vi "SaveImg.vi"(0 "零件型号":string, 1 "Image":T1, 2 "Fold路径":path) -> ()   [LabVIEW 2014]
uses:
  <vilib>/vision/Image Controls.llb/IMAQ Image.ctl
panel:
  out "添加的路径":path
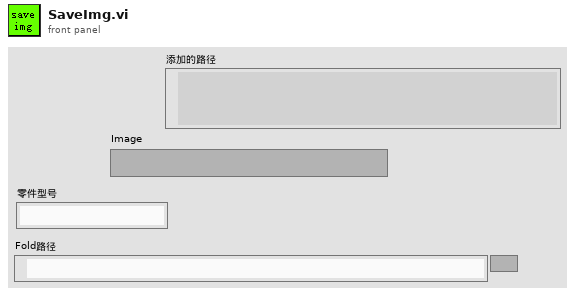
[diagram p1: front panel]
types:
  T1 = typedef "IMAQ Image.ctl" = refnum<image>
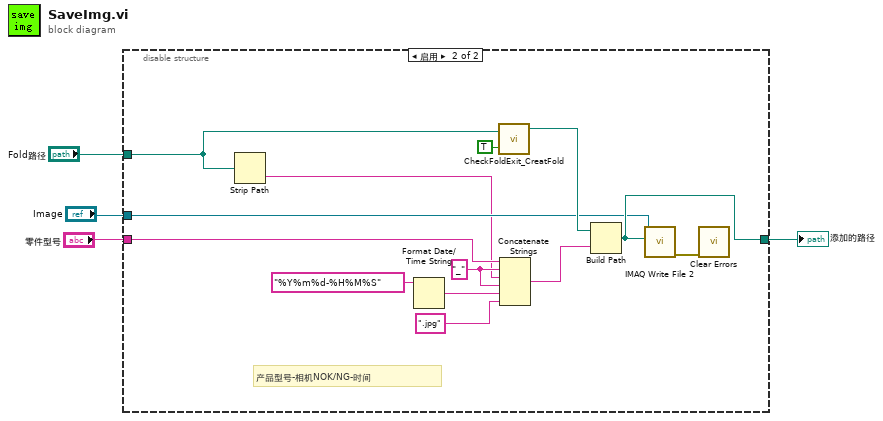
[diagram p0: block diagram]
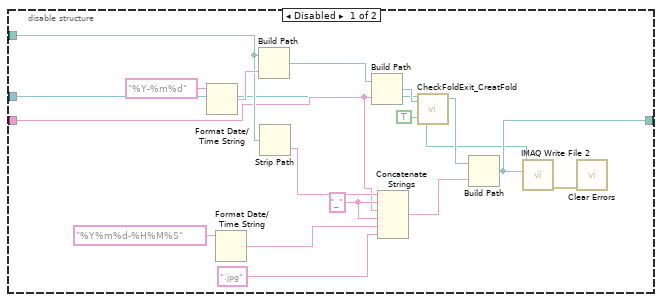
[diagram p2: hidden frame]
diagram:
  n1 = disable-structure shown="启用" {
    disable-tunnel: [w18 w26] -> w4
    disable-tunnel: "Fold路径" -> [w9 w22]
    disable-tunnel: "零件型号" -> [w6 w24]
    disable-tunnel: "Image" -> [w5 w25]
    frame Disabled {
      w7 = "_" ("字符串")
      n2 = Format Date/Time String(time format string (%c)="%Y-%m%d") -> (date/time string=w21:string)  [unwired: 2 in]
      n3 = Format Date/Time String(time format string (%c)="%Y%m%d-%H%M%S") -> (date/time string=w16:string)  [unwired: 2 in]
      n4 = Build Path(base path=w9, name or relative path=w21) -> (appended path=w10:path)
      n5 = Strip Path(path=w9) -> (name=w8:string)  [unwired: 1 out]
      n6 = Build Path(base path=w10, name or relative path=w6) -> (appended path=w12:path)
      n7 = Concatenate Strings(w8, w7, w6, w7, w16, ".jpg" ("string")) -> (w17:string)
      n8 = call "CheckFoldExit_CreatFold.vi"("path in"=w12, "FoldOrFile¡H"=TRUE) -> ("File out"=w11:path)  [unwired: 2 out]
      n9 = Build Path(base path=w11, name or relative path=w17) -> (appended path=w18:path)
      n10 = call-poly "IMAQ Write File 2"("File Path"=w18, "Image"=w5) -> ("error out"=w14:errorcluster)  [unwired: 8 in, 1 out]
      n11 = call <vilib>:"Clear Errors.vi"("error in (no error)"=w14) -> ()  [unwired: 5 in, 2 out]
    }
    frame Enabled {
      w34 = "_" ("字符串")
      # "产品型号-相机NOK/NG-时间"
      n12 = Strip Path(path=w22) -> (name=w23:string)  [unwired: 1 out]
      n13 = Format Date/Time String(time format string (%c)="%Y%m%d-%H%M%S") -> (date/time string=w29:string)  [unwired: 2 in]
      n14 = call "CheckFoldExit_CreatFold.vi"("path in"=w22, "FoldOrFile¡H"=TRUE) -> ("File out"=w33:path)  [unwired: 2 out]
      n15 = Concatenate Strings(w24, w34, w23, w34, w29, ".jpg" ("string")) -> (w28:string)
      n16 = Build Path(base path=w33, name or relative path=w28) -> (appended path=w26:path)
      n17 = call-poly "IMAQ Write File 2"("File Path"=w26, "Image"=w25) -> ("error out"=w31:errorcluster)  [unwired: 8 in, 1 out]
      n18 = call <vilib>:"Clear Errors.vi"("error in (no error)"=w31) -> ()  [unwired: 5 in, 2 out]
    }
  }
  "添加的路径" <- w4
